vi "Get Sheet by Index.vi"(8 "error in (no error)":errorcluster, 10 "Sheet Index":i32, 11 "Excel Interface in":refnum<class "Excel Interface.lvclass">) -> (0 "error out":errorcluster, 2 "Excel Sheet out":refnum<class "Excel Sheet.lvclass">, 3 "Excel Interface out":refnum<class "Excel Interface.lvclass">)   [LabVIEW 2016, in "Excel Interface.lvclass"]
uses:
  Excel Interface.lvclass
  Excel Sheet/Excel Sheet.lvclass
  Excel Interface.lvclass/Excel Interface.ctl
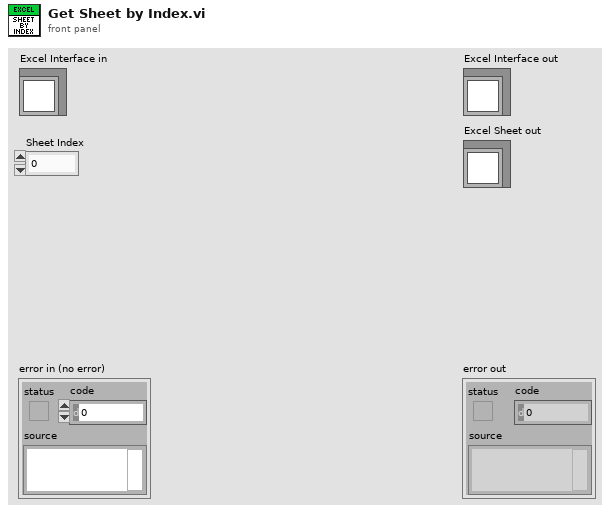
[diagram p1: front panel]
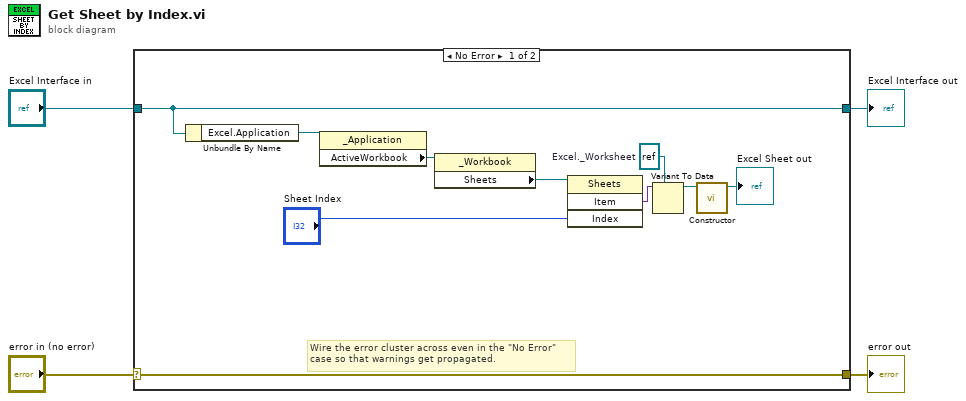
[diagram p0: block diagram]
diagram:
  n1 = case shown="No Error" "error in (no error)" {
    selector: "error in (no error)" -> [w14 w16]
    tunnel: [w14 w16] -> w3
    tunnel: [w13 w15] -> w1
    tunnel: "Excel Interface in" -> [w13 w15]
    frame No Error {
      w7 = refnum<k7> refnum  # Excel._Worksheet
      # "Wire the error cluster across even in the \"No Error\"\ncase so that warnings get propagated."
      n2 = Unbundle By Name(w13) -> ("Excel.Application"=w12:refnum<k7>)
      n3 = property class="_Application"(reference=w12) -> ("ActiveWorkbook"=w11:refnum<k7>)  [unwired: 1 in, 2 out]
      n4 = property class="_Workbook"(reference=w11) -> ("Sheets"=w10:refnum<k7>)  [unwired: 1 in, 2 out]
      n5 = invoke class="Sheets" method="Item"(reference=w10, "Index"="Sheet Index") -> ("Item"=w8:variant)  [unwired: 2 in, 3 out]
      n6 = Variant To Data(type=w7, Variant=w8) -> (data=w6:refnum<k7>)  [unwired: 1 in, 1 out]
      n7 = call "Constructor.vi"("Worksheet"=w6) -> ("Excel Sheet out"=→"Excel Sheet out":refnum<class "Excel Sheet.lvclass">)  [unwired: 10 in]
    }
    frame Error {
    }
  }
  "error out" <- w3
  "Excel Interface out" <- w1
